vi "MessdatenSchreiben.vi"(10 "Waveform":waveform(dbl), 11 "Byte Stream File in":refnum<file>) -> (0 "error out":errorcluster, 3 "Byte Stream File out":refnum<file>)   [LabVIEW 2023]
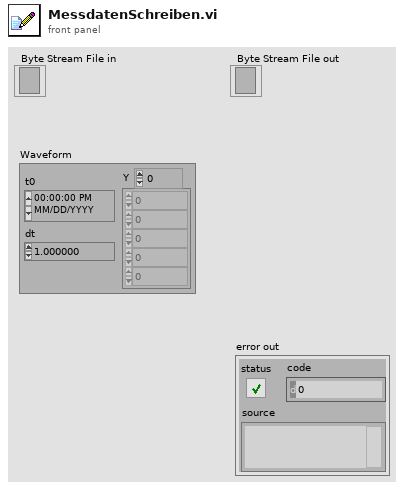
[diagram p1: front panel]
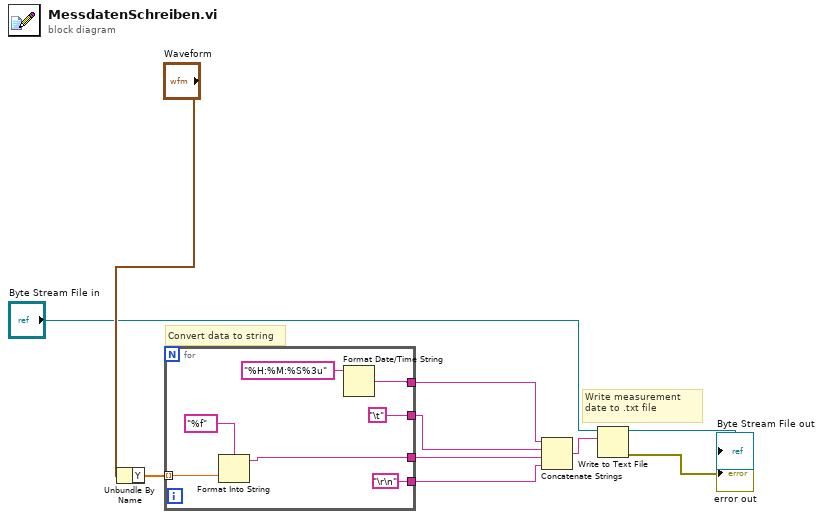
[diagram p0: block diagram]
diagram:
  # "Convert data to string"
  # "Write measurement date to .txt file"
  n1 = Unbundle By Name("Waveform") -> ("Y"=w4:dbl[])
  n2 = for {
    tunnel: [w16] -> w5
    tunnel: w4 -> [w15] mode=indexing
    tunnel: [w12] -> w3
    tunnel: ["\t" ("Tab")] -> w2
    tunnel: ["\r\n"] -> w1
    n3 = Format Into String(format string="%f", w15) -> (resulting string=w16:string)  [unwired: 2 in, 1 out]
    n4 = Format Date/Time String(time format string (%c)="%H:%M:%S%3u") -> (date/time string=w12:string)  [unwired: 2 in]
  }
  n5 = Concatenate Strings(w3, w2, w5, w1) -> (w6:string)
  n6 = Write to Text File(file (use dialog)="Byte Stream File in", text=w6) -> (refnum out=→"Byte Stream File out":refnum<file>, error out=→"error out":errorcluster)  [unwired: 2 in, 1 out]
